vi "IN_RANGE_CHECKING.vi"(8 "error in (no error)":errorcluster, 10 "Load Cell Scaned":string, 11 "AUTO CYC DATA in":T2) -> (0 "error out":errorcluster, 2 "Cluster":cluster{dbl[], dbl[]}, 3 "AUTO CYC DATA out":T2, 5 "Enum":T1=enum."TRIP FORCE HIGHER FAIL")   [LabVIEW 2017]
uses:
  Controls/AUTO_DATA.ctl
  Controls/TRIP_VALUS_STATUS.ctl
  <userlib>/_OpenG.lib/array/array.llb/Sort 1D Array (DBL)__ogtk.vi
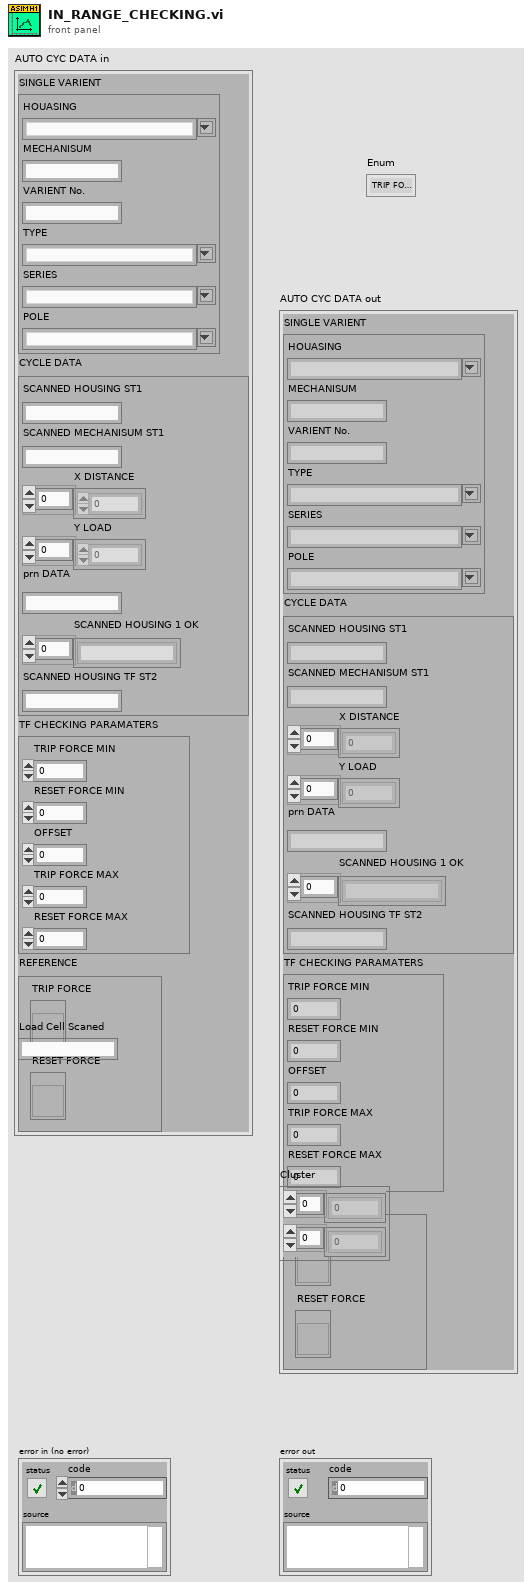
[diagram p1: front panel]
types:
  T1 = typedef "TRIP_VALUS_STATUS.ctl" = enum16{"RESET FORCE HIGHER FAIL", "TRIP FORCE HIGHER FAIL", "TRIP FORCE LOWER FAIL", "IDEAL", "TRIP RESET ACHIVED"}
  T2 = typedef "AUTO_DATA.ctl" = cluster{"SINGLE VARIENT":cluster{"HOUASING":string, "MECHANISUM":string, "VARIENT No.":string, "TYPE":string, "SERIES":string, "POLE":string}, "CYCLE DATA":cluster{"SCANNED HOUSING ST1":string, "SCANNED MECHANISUM ST1":string, "X DISTANCE":dbl[], "Y LOAD":dbl[], "prn DATA":string, "SCANNED HOUSING 1 OK":string[], "SCANNED HOUSING TF ST2":string}, "TF CHECKING PARAMATERS":cluster{"TRIP FORCE MIN":u16, "RESET FORCE MIN":u16, "OFFSET":i16, "TRIP FORCE MAX":u16, "RESET FORCE MAX":u16}, "REFERENCE":cluster{"TRIP FORCE":refnum<vi>, "RESET FORCE":refnum<vi>}}
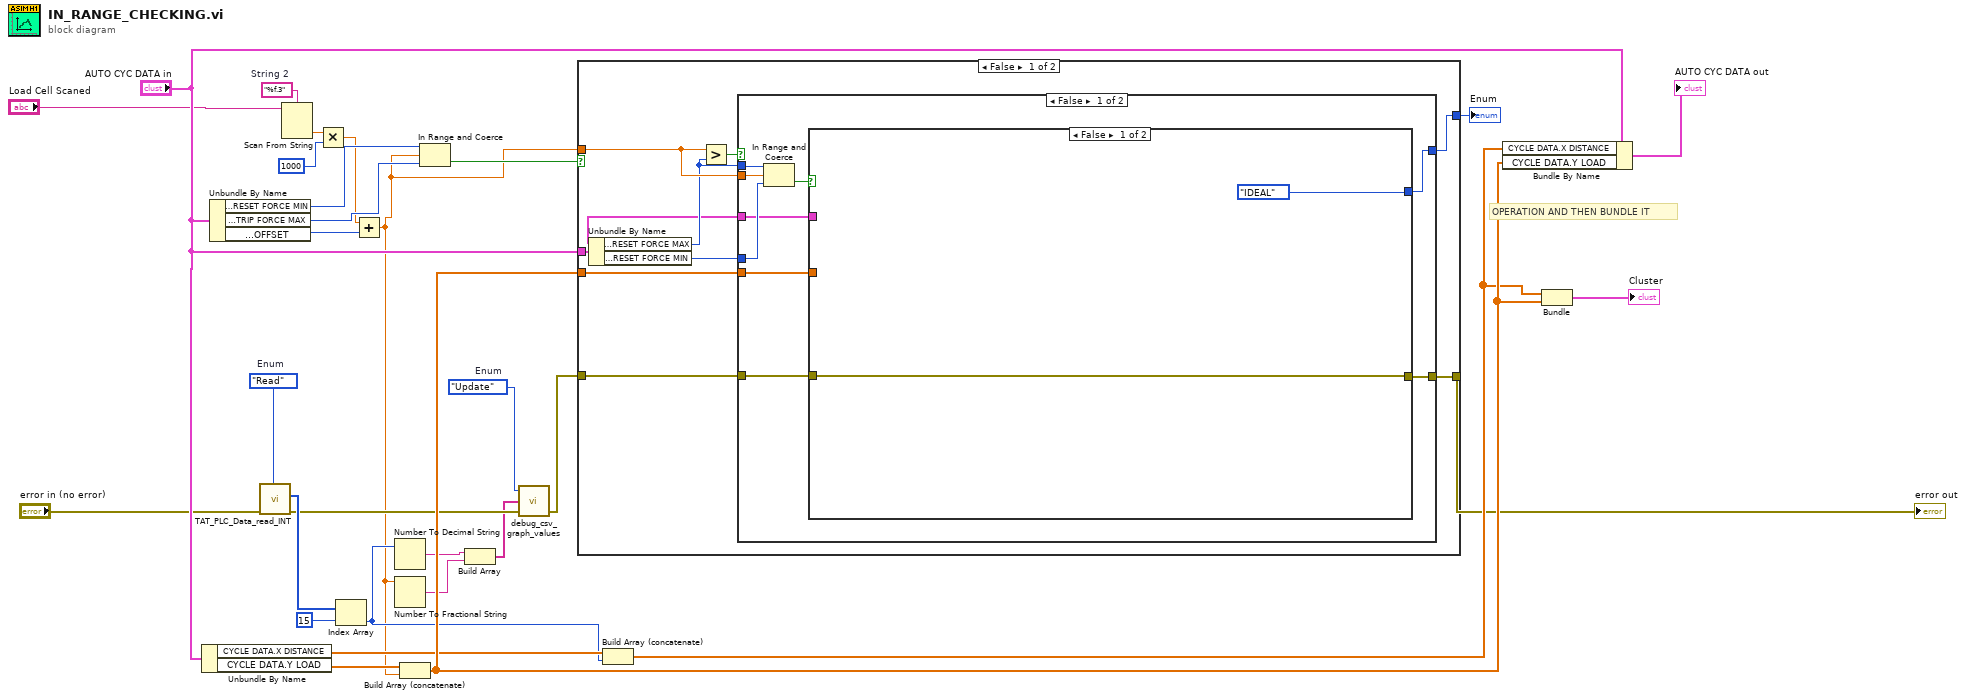
[diagram p0: block diagram]
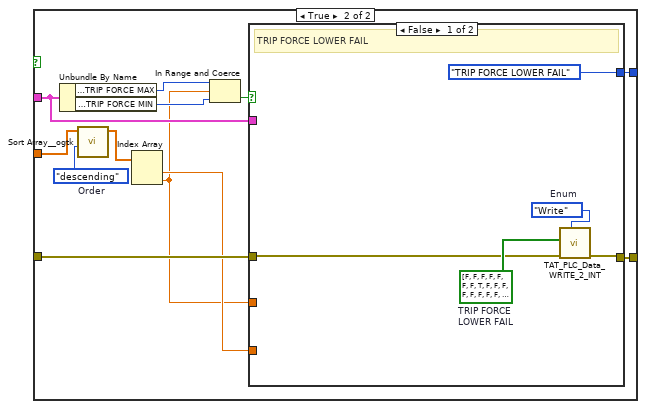
[diagram p2: hidden frame]
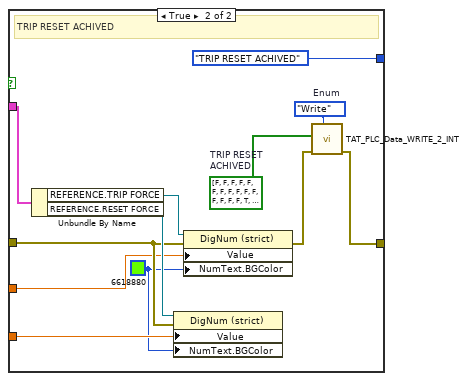
[diagram p3: hidden frame]
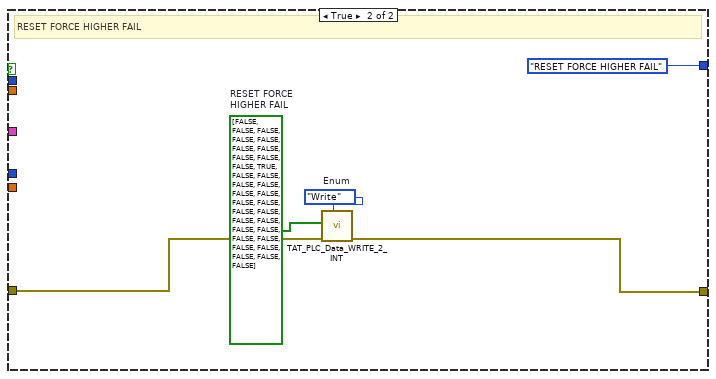
[diagram p4: hidden frame]
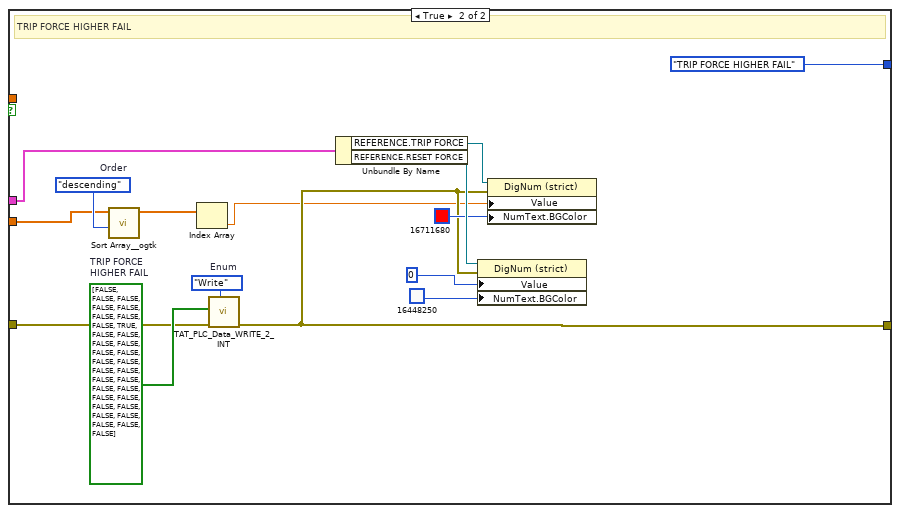
[diagram p5: hidden frame]
diagram:
  w9 = enum16{"Int", "Update"}."Update"  # Enum
  w19 = "%f.3"  # String 2
  w13 = enum16{"Read", "Write"}."Read"  # Enum
  # "OPERATION AND THEN BUNDLE IT"
  n1 = Unbundle By Name("AUTO CYC DATA in") -> ("CYCLE DATA.X DISTANCE"=w27:dbl[], "CYCLE DATA.Y LOAD"=w28:dbl[])
  n2 = Unbundle By Name("AUTO CYC DATA in") -> ("TF CHECKING PARAMATERS.RESET FORCE MIN"=w25:u16, "TF CHECKING PARAMATERS.TRIP FORCE MAX"=w26:u16, "TF CHECKING PARAMATERS.OFFSET"=w11:i16)
  n3 = call "TAT_PLC_Data_read_INT.vi"("Enum"=w13, "error in (no error)"="error in (no error)") -> ("error out"=w8:errorcluster, "Array 2"=w12:u16[])  [unwired: 8 in]
  n4 = Scan From String(format string=w19, input string="Load Cell Scaned") -> (output 1=w20:dbl)  [unwired: 3 in, 3 out]
  n5 = Multiply(x=w20, y=1000) -> (x*y=w22:dbl)
  n6 = Index Array(array=w12, index=15) -> (element=w5:u16)
  n7 = Add(x=w22, y=w11) -> (x+y=w2:dbl)
  n8 = Number To Decimal String(number=w5) -> (decimal integer string=w4:string)  [unwired: 1 in]
  n9 = Number To Fractional String(number=w2) -> (F-format string=w6:string)  [unwired: 3 in]
  n10 = Build Array (concatenate)(w28, w2) -> (w30:dbl[])
  n11 = In Range and Coerce(upper limit=w25, x=w2, lower limit=w26) -> (In Range?=w24:bool)  [unwired: 1 out]
  n12 = Build Array(w4, w6) -> (w3:string[])
  n13 = call "debug_csv_graph_values.vi"("error in"=w8, "Value Distance/Load"=w3, "Enum"=w9) -> ("error our"=w7:errorcluster)  [unwired: 1 in, 1 out]
  n14 = case shown="False" w24 {
    tunnel: w2 -> [w38 _]
    tunnel: "AUTO CYC DATA in" -> [w34 w93]
    tunnel: w30 -> [w35 w87]
    tunnel: w7 -> [w33 w97]
    tunnel: [w32 w92] -> w10
    tunnel: [w31 TRIP_VALUS_STATUS."TRIP FORCE HIGHER FAIL"] -> w1
    frame False {
      n15 = Unbundle By Name(w34) -> ("TF CHECKING PARAMATERS.RESET FORCE MAX"=w37:u16, "TF CHECKING PARAMATERS.RESET FORCE MIN"=w36:u16)
      n16 = Greater?(x=w38, y=w37) -> (0:w39:bool)
      n17 = case shown="False" w39 {
        tunnel: w38 -> [w48 _]
        tunnel: w37 -> [w47 _]
        tunnel: w36 -> [w46 _]
        tunnel: w35 -> [w44 _]
        tunnel: w34 -> [w43 _]
        tunnel: w33 -> [w42 w82]
        tunnel: [w41 w81] -> w32
        tunnel: [w40 TRIP_VALUS_STATUS."RESET FORCE HIGHER FAIL"] -> w31
        frame False {
          n18 = In Range and Coerce(upper limit=w47, x=w48, lower limit=w46) -> (In Range?=w45:bool)  [unwired: 1 out]
          n19 = case shown="False" w45 {
            tunnel: w44 -> [_ w60]
            tunnel: w43 -> [_ w54]
            tunnel: w42 -> [w50 w56]
            tunnel: [w50 w55] -> w41
            tunnel: [TRIP_VALUS_STATUS."IDEAL" w51] -> w40
            frame False {
            }
            frame True {
              w62 = enum16{"ascending", "descending"}."descending"  # Order
              n20 = Unbundle By Name(w54) -> ("TF CHECKING PARAMATERS.TRIP FORCE MAX"=w59:u16, "TF CHECKING PARAMATERS.TRIP FORCE MIN"=w58:u16)
              n21 = call-poly <userlib>:"Sort Array__ogtk.vi"("Order"=w62, "Array in"=w60) -> ("Sorted Array out"=w61:dbl[])  [unwired: 8 in, 1 out]
              n22 = Index Array(array=w61) -> (element #1=w53:dbl, element #2=w52:dbl)  [unwired: 2 in]
              n23 = In Range and Coerce(upper limit=w59, x=w52, lower limit=w58) -> (In Range?=w57:bool)  [unwired: 1 out]
              n24 = case shown="False" w57 {
                tunnel: w56 -> [w65 w72]
                tunnel: [w64 w77] -> w55
                tunnel: w54 -> [_ w76]
                tunnel: w53 -> [_ w71]
                tunnel: w52 -> [_ w70]
                tunnel: [TRIP_VALUS_STATUS."TRIP FORCE LOWER FAIL" TRIP_VALUS_STATUS."TRIP RESET ACHIVED"] -> w51
                frame False {
                  w67 = bool[] [FALSE, FALSE, FALSE, FALSE, FALSE, FALSE, FALSE, TRUE, FALSE, FALSE, FALSE, FALSE, FALSE, FALSE, FALSE, FALSE, FALSE, FALSE, FALSE, FALSE, FALSE, FALSE, FALSE, FALSE, FALSE, FALSE, FALSE, FALSE, FALSE, FALSE, FALSE, FALSE]  # TRIP FORCE LOWER FAIL
                  w66 = enum16{"Read", "Write"}."Write"  # Enum
                  # "TRIP FORCE LOWER FAIL"
                  n25 = call "TAT_PLC_Data_WRITE_2_INT.vi"("Enum"=w66, "error in (no error)"=w65, "Array"=w67) -> ("error out"=w64:errorcluster)  [unwired: 7 in, 1 out]
                }
                frame True {
                  w69 = u32 6618880
                  w78 = bool[] [FALSE, FALSE, FALSE, FALSE, FALSE, FALSE, FALSE, FALSE, FALSE, FALSE, FALSE, FALSE, FALSE, FALSE, FALSE, TRUE, FALSE, FALSE, FALSE, FALSE, FALSE, FALSE, FALSE, FALSE, FALSE, FALSE, FALSE, FALSE, FALSE, FALSE, FALSE, FALSE]  # TRIP RESET ACHIVED
                  w79 = enum16{"Read", "Write"}."Write"  # Enum
                  # "TRIP RESET ACHIVED"
                  n26 = Unbundle By Name(w76) -> ("REFERENCE.TRIP FORCE"=w74:refnum<vi>, "REFERENCE.RESET FORCE"=w73:refnum<vi>)
                  n27 = property on="Property Node" class="DigNum (strict)"(reference=w73, error in=w72, "Value"=w71, "NumText.BGColor"=w69) -> ()  [unwired: 2 out]
                  n28 = property on="Property Node" class="DigNum (strict)"(reference=w74, error in=w72, "Value"=w70, "NumText.BGColor"=w69) -> (error out=w75:errorcluster)  [unwired: 1 out]
                  n29 = call "TAT_PLC_Data_WRITE_2_INT.vi"("Enum"=w79, "error in (no error)"=w75, "Array"=w78) -> ("error out"=w77:errorcluster)  [unwired: 7 in, 1 out]
                }
              }
            }
          }
        }
        frame True {
          w83 = bool[] [FALSE, FALSE, FALSE, FALSE, FALSE, FALSE, FALSE, FALSE, FALSE, FALSE, TRUE, FALSE, FALSE, FALSE, FALSE, FALSE, FALSE, FALSE, FALSE, FALSE, FALSE, FALSE, FALSE, FALSE, FALSE, FALSE, FALSE, FALSE, FALSE, FALSE, FALSE, FALSE]  # RESET FORCE HIGHER FAIL
          w84 = enum16{"Read", "Write"}."Write"  # Enum
          # "RESET FORCE HIGHER FAIL"
          n30 = call "TAT_PLC_Data_WRITE_2_INT.vi"("Enum"=w84, "error in (no error)"=w82, "Array"=w83) -> ("error out"=w81:errorcluster)  [unwired: 7 in, 1 out]
        }
      }
    }
    frame True {
      w88 = enum16{"ascending", "descending"}."descending"  # Order
      w98 = bool[] [FALSE, FALSE, FALSE, FALSE, FALSE, FALSE, FALSE, FALSE, TRUE, FALSE, FALSE, FALSE, FALSE, FALSE, FALSE, FALSE, FALSE, FALSE, FALSE, FALSE, FALSE, FALSE, FALSE, FALSE, FALSE, FALSE, FALSE, FALSE, FALSE, FALSE, FALSE, FALSE]  # TRIP FORCE HIGHER FAIL
      w99 = enum16{"Read", "Write"}."Write"  # Enum
      # "TRIP FORCE HIGHER FAIL"
      n31 = call-poly <userlib>:"Sort Array__ogtk.vi"("Order"=w88, "Array in"=w87) -> ("Sorted Array out"=w86:dbl[])  [unwired: 8 in, 1 out]
      n32 = Index Array(array=w86) -> (element=w90:dbl)  [unwired: 1 in]
      n33 = call "TAT_PLC_Data_WRITE_2_INT.vi"("Enum"=w99, "error in (no error)"=w97, "Array"=w98) -> ("error out"=w92:errorcluster)  [unwired: 7 in, 1 out]
      n34 = Unbundle By Name(w93) -> ("REFERENCE.TRIP FORCE"=w96:refnum<vi>, "REFERENCE.RESET FORCE"=w95:refnum<vi>)
      n35 = property on="Property Node" class="DigNum (strict)"(reference=w95, error in=w92, "Value"=0, "NumText.BGColor"=u32 16448250) -> ()  [unwired: 2 out]
      n36 = property on="Property Node" class="DigNum (strict)"(reference=w96, error in=w92, "Value"=w90, "NumText.BGColor"=u32 16711680) -> ()  [unwired: 2 out]
    }
  }
  "error out" <- w10
  "Enum" <- w1
  n37 = Build Array (concatenate)(w27, w5) -> (w17:dbl[])
  n38 = Bundle By Name(cluster="AUTO CYC DATA in", "CYCLE DATA.X DISTANCE"=w17, "CYCLE DATA.Y LOAD"=w30) -> (→"AUTO CYC DATA out":T2)
  n39 = Bundle(w17, w30) -> (→"Cluster":cluster{dbl[], dbl[]})  [unwired: 1 in]
